vi "JSON Schema to Table.vi"(8 "error in (no error)":errorcluster, 11 "JSON Schema in":string) -> (0 "error out":errorcluster, 2 "Table":string[][](table), 3 "JSON Schema out":string)   [LabVIEW 2019, in "JSON-Schema.lvlib"]
doc: "Represent <b>JSON Schema in</b> as a table of JSON Schema keywords."
uses:
  JSON-Schema.lvlib
  a58aa99b-14ca-48af-b081-8c0a9da57a3d.vi
  fd2d87a8-6ab4-473d-a4e8-527c74bc07ef.vi
  <vilib>/JDP Science/JSONtext/Next JSON Value.vi
  <vilib>/JDP Science/JSONtext/String Subset.vi
  <vilib>/JDP Science/JSONtext/Parsing/Advance past next JSON Value (inlined COPY).vi
  <vilib>/JDP Science/JSONtext/Parsing/Advance past whitespace.vi
  <vilib>/JDP Science/JSONtext/Parsing/Advance past String.vi
  <vilib>/JDP Science/JSONtext/Parsing/Advance past Number.vi
  <vilib>/JDP Science/JSONtext/Parsing/Advance past Line Ending.vi
  <vilib>/JDP Science/JSONtext/Parsing/Parse Full Path or Item Name.vi
  <vilib>/JDP Science/JSONtext/Parsing/Advance past Array.vi
  <vilib>/JDP Science/JSONtext/Parsing/Advance past Object.vi
  <vilib>/JDP Science/JSONtext/support/Error Cluster From Code.vi
  <vilib>/JDP Science/JSONtext/Offset/Find Item Locations by Path.vi
  <vilib>/JDP Science/JSONtext/JSON text to Variant.vi
  <vilib>/JDP Science/JSONtext/LVClass Serializer/JSONtext LVClass Serializer.lvclass
  <vilib>/JDP Science/JSONtext/JSONtext.lvlib
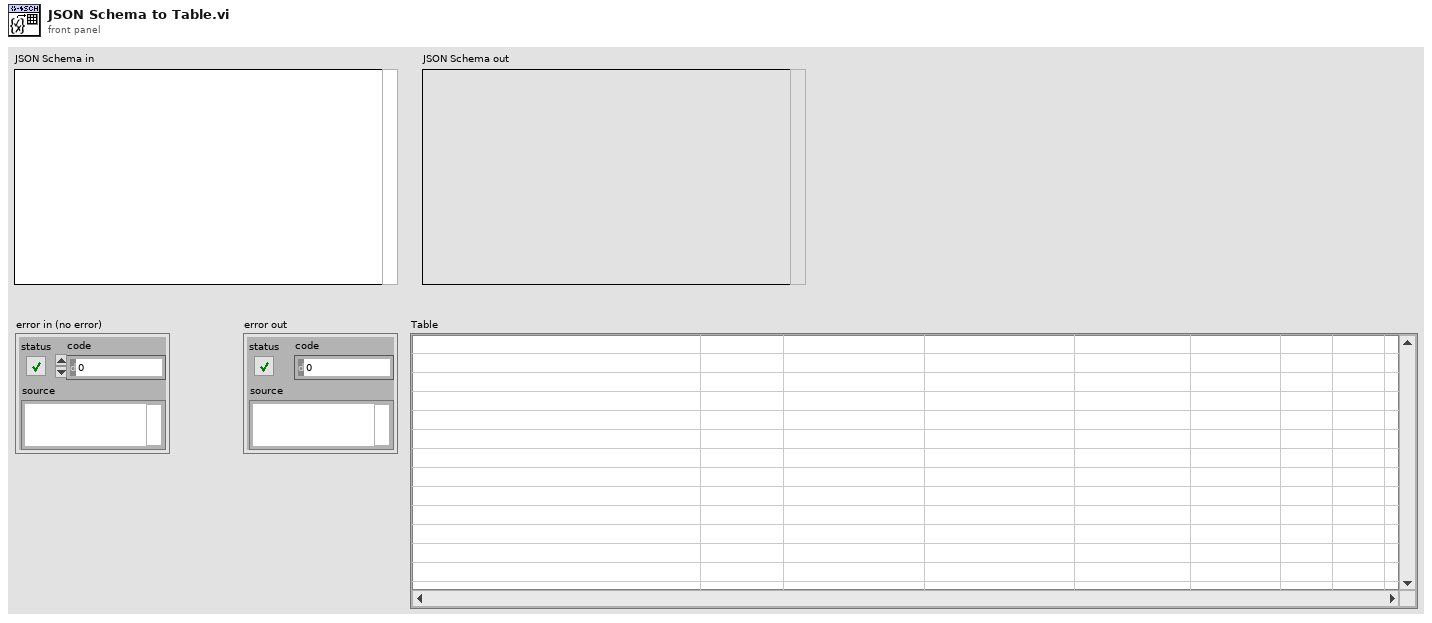
[diagram p1: front panel]
types:
  T1 = typedef "JSONtext.lvlib/JSON Value Type.ctl" = enum16{"Not a JSON Value", "JSON Object", "JSON Array", "String", "Number", "true", "false", "null"}
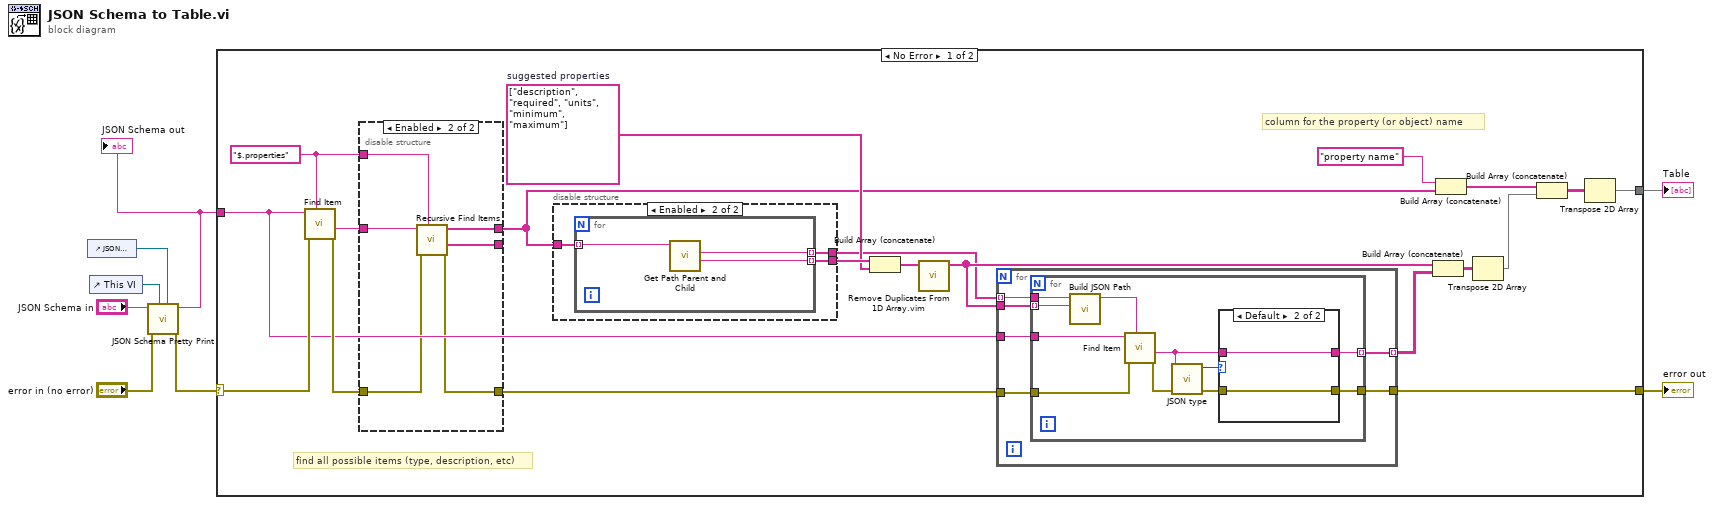
[diagram p0: block diagram]
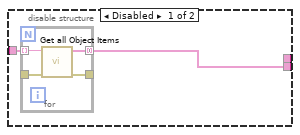
[diagram p2: hidden frame]
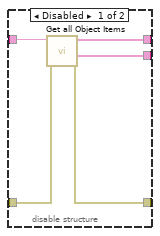
[diagram p3: hidden frame]
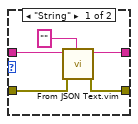
[diagram p4: hidden frame]
diagram:
  n1 = control-ref of="JSON Schema out"() -> (w5:refnum<vi>)
  n2 = control-ref of="This VI"() -> (w6:refnum<vi>)
  n3 = call "JSON Schema Pretty Print.vi"("String Control"=w5, "reference"=w6, "error in (no error)"="error in (no error)", "<JSON> in"="JSON Schema in") -> ("error out"=w3:errorcluster, "<JSON> out"=w1:string)  [unwired: 6 in]
  "JSON Schema out" <- w1
  n4 = case shown="No Error" w3 {
    selector: w3 -> [w28 w75]
    tunnel: w1 -> [w9 _]
    tunnel: [w23 _] -> w8
    tunnel: [w21 w75] -> w7
    frame No Error {
      w16 = string[] ["description", "required", "units", "minimum", "maximum"]  # suggested properties
      w15 = "$.properties" ("$Path or Item Name")
      # "column for the property (or object) name"
      # "find all possible items (type, description, etc)"
      n5 = call <vilib>:"Find Item.vi"("$Path or Item Name"=w15, "error in (no error)"=w28, "JSON"=w9) -> ("error out"=w22:errorcluster, "<JSON>"=w10:string)  [unwired: 5 in, 2 out]
      n6 = disable-structure shown="Enabled" {
        disable-tunnel: w10 -> [w45 w51]
        disable-tunnel: w22 -> [w44 w50]
        disable-tunnel: [w43 w48] -> w11
        disable-tunnel: [w42 w47] -> _
        disable-tunnel: [w41 w49] -> w14
        disable-tunnel: w15 -> [_ w46]
        frame Disabled {
          n7 = call <vilib>:"Get all Object Items.vi"("error in (no error)"=w44, "JSON"=w45) -> ("error out"=w41:errorcluster, "<JSON>"=w42:string[], "Item Names"=w43:string[])  [unwired: 6 in, 1 out]
        }
        frame Enabled {
          n8 = call "Recursive Find Items.vi"("$Path or Item Name"=w46, "error in (no error)"=w50, "JSON Schema in"=w51) -> ("error out"=w49:errorcluster, "<JSON> Items"=w47:string[], "Item Names"=w48:string[])  [unwired: 5 in, 1 out]
        }
      }
      n9 = disable-structure shown="Enabled" {
        disable-tunnel: [w30 w36] -> w17
        disable-tunnel: w11 -> [w29 w37]
        disable-tunnel: [_ w35] -> w13
        frame Disabled {
          n10 = for {
            tunnel: w29 -> [w34] mode=indexing
            tunnel: [w33] -> w30 mode=concatenating
            tunnel: _ -> [w32]
            tunnel: [w31] -> _
            n11 = call <vilib>:"Get all Object Items.vi"("error in (no error)"=w32, "JSON"=w34) -> ("error out"=w31:errorcluster, "Item Names"=w33:string[])  [unwired: 6 in, 2 out]
          }
        }
        frame Enabled {
          n12 = for {
            tunnel: w37 -> [w40] mode=indexing
            tunnel: [w39] -> w36 mode=indexing
            tunnel: [w38] -> w35 mode=indexing
            n13 = call "Get Path Parent and Child.vi"("$Path"=w40) -> ("Child"=w39:string, "$.Parent"=w38:string)  [unwired: 8 in, 1 out]
          }
        }
      }
      n14 = Build Array (concatenate)(w17, w16) -> (w18:string[])
      n15 = call "Remove Duplicates From 1D Array.vim"("array"=w18) -> ("array with duplicates removed"=w20:string[])  [unwired: 10 in]
      n16 = for {
        tunnel: w9 -> [w57]
        tunnel: w20 -> [w56]
        tunnel: [w55] -> w24 mode=indexing
        tunnel: w14 -> [w54]
        tunnel: [w53] -> w21
        tunnel: w13 -> [w52] mode=indexing
        n17 = for {
          tunnel: w57 -> [w67]
          tunnel: w56 -> [w59] mode=indexing
          tunnel: [w65] -> w55 mode=indexing
          tunnel: w54 -> [w62]
          tunnel: [w61] -> w53
          tunnel: w52 -> [w58]
          n18 = call "Build JSON Path.vi"("Child element"=w59, "Base $Path"=w58) -> ("$Path out"=w60:string)  [unwired: 9 in]
          n19 = call <vilib>:"Find Item.vi"("$Path or Item Name"=w60, "error in (no error)"=w62, "JSON"=w67) -> ("error out"=w63:errorcluster, "<JSON>"=w64:string)  [unwired: 5 in, 2 out]
          n20 = call <vilib>:"JSON type.vi"("JSON"=w64) -> ("JSON Value Type"=w66:T1)  [unwired: 9 in, 1 out]
          n21 = case shown="Default" w66 {
            tunnel: [w72 w74] -> w65
            tunnel: w64 -> [w70 w74]
            tunnel: w63 -> [w69 w73]
            tunnel: [w68 w73] -> w61
            frame "String" {
              n22 = call "From JSON Text.vim"("Data Type and Default Value"="", "error in (no error)"=w69, "JSON"=w70) -> ("error out"=w68:errorcluster, "Data out"=w72:string)  [unwired: 7 in]
            }
            frame Default {
            }
          }
        }
      }
      n23 = Build Array (concatenate)(w20, w24) -> (w25:string[][])
      n24 = Build Array (concatenate)("property name" ("$Path or Item Name"), w11) -> (w19:string[])
      n25 = Transpose 2D Array(2D array=w25) -> (transposed array=w12:string[][])
      n26 = Build Array (concatenate)(w19, w12) -> (w26:string[][])
      n27 = Transpose 2D Array(2D array=w26) -> (transposed array=w23:string[][])
    }
    frame Error {
    }
  }
  "Table" <- w8
  "error out" <- w7
